vi "TCP_initDriver.vi"(10 "address":string="192.168.24.142", 11 "remote port or service name":u16=7776) -> (0 "error out":errorcluster, 2 "Driver Response":bool, 3 "TCP Network Connection out":refnum<k5>)   [LabVIEW 2019]
panel:
  in  "Set_Velocity":dbl=0.5
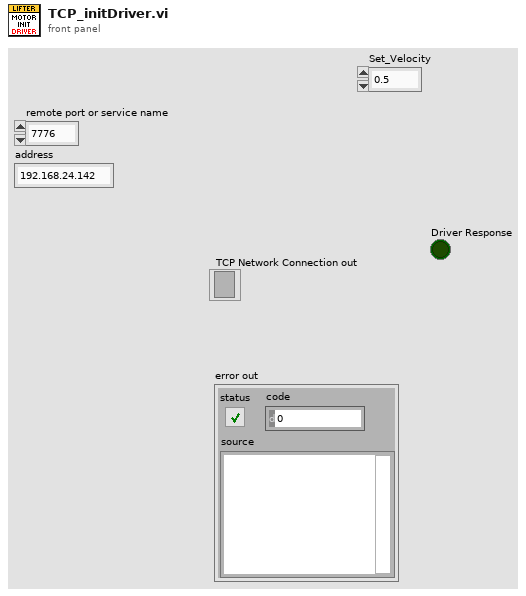
[diagram p1: front panel]
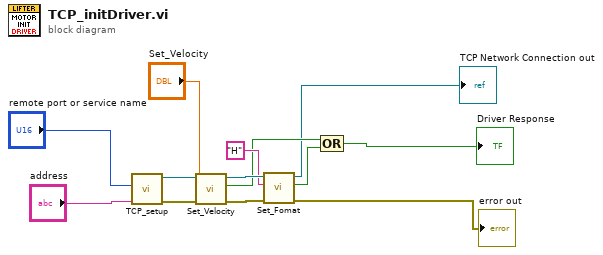
[diagram p0: block diagram]
diagram:
  n1 = call "TCP_setup.vi"("address"="address", "remote port or service name"="remote port or service name") -> ("error out"=w4:errorcluster, "TCP Network Connection out"=w5:refnum<k5>)  [unwired: 8 in]
  n2 = call "Set_Velocity.vi"("error in (no error)"=w4, "Set_Velocity"="Set_Velocity", "connection ID"=w5) -> ("error out"=w12:errorcluster, "Driver response"=w10:bool, "TCP Network Connection out"=w13:refnum<k5>)  [unwired: 6 in]
  n3 = call "Set_Fomat.vi"("error in (no error)"=w12, "Parameter 2"="H", "connection ID"=w13) -> ("error out"=→"error out":errorcluster, "Driver response"=w9:bool, "TCP Network Connection out"=→"TCP Network Connection out":refnum<k5>)  [unwired: 6 in]
  n4 = Compound Arithmetic op=OR(w10, w9) -> (→"Driver Response":bool)
